vi "Write remote_address .vi"(8 "error in (no error)":errorcluster, 10 "remote_address":string, 11 "Socket.TCP in":refnum<class "Socket.TCP.lvclass">) -> (0 "error out":errorcluster, 3 "Socket.TCP out":refnum<class "Socket.TCP.lvclass">)   [LabVIEW 2014, in "Socket.lvlib" / "Socket.TCP.lvclass"]
uses:
  Socket.TCP.lvclass
  Socket.TCP.lvclass/Socket.TCP.ctl
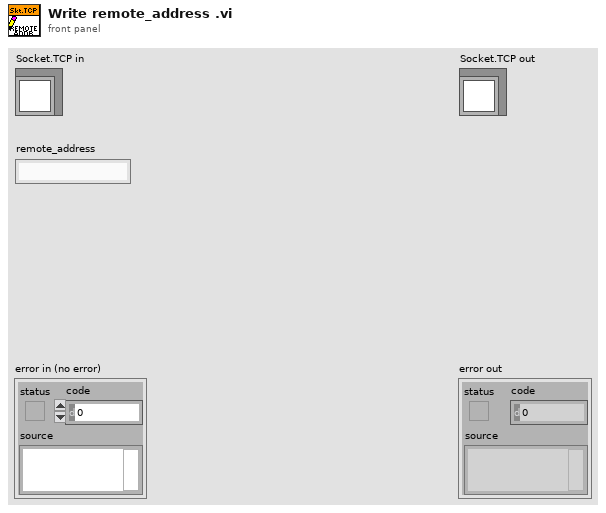
[diagram p1: front panel]
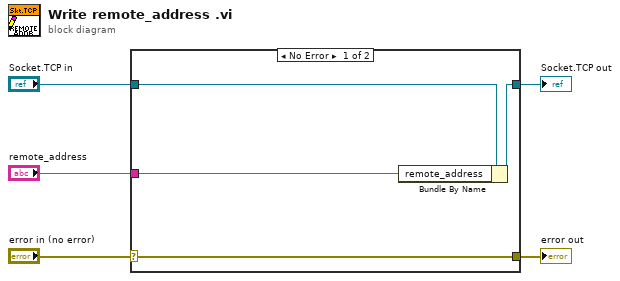
[diagram p0: block diagram]
diagram:
  n1 = case shown="No Error" "error in (no error)" {
    selector: "error in (no error)" -> [w9 w10]
    tunnel: [w9 w10] -> w4
    tunnel: [w7 w11] -> w2
    tunnel: "Socket.TCP in" -> [w8 w11]
    tunnel: "remote_address" -> [w6 _]
    frame No Error {
      n2 = Bundle By Name(cluster=w8, "remote_address"=w6) -> (w7:refnum<class "Socket.TCP.lvclass">)
    }
    frame Error {
    }
  }
  "error out" <- w4
  "Socket.TCP out" <- w2
